vi "MeasurementSMO.TestLauncher.vi"() -> ()   [LabVIEW 2019, in "MeasurementSMO.lvclass"]
uses:
  MeasurementSMO.lvclass
  <vilib>/JKI/JKI SMO/SMO/SMO.lvclass
  <vilib>/JKI/JKI SMO/SMO/Typedefs/SMOState --Enum.ctl
  <userlib>/LevyLab/Instrument Framework/SMOs/RemoteControl/RemoteControl.lvclass
  <userlib>/LevyLab/Instrument Framework/SMOs/RemoteControl/Typedefs/RC Com Type--enum.ctl
  21cc0d15-aa5c-4e02-9f98-410864ffd08d.vi
  2cee4e23-403c-4d2f-920d-9f09caed685e.vi
  9af032d4-89d2-4663-9556-aa01e6123ab8.vi
  C:/Program Files (x86)/National Instruments/LabVIEW 2019/vi.lib/JKI/JKI SMO/SMO/SMO.lvclass
  b9372eaf-d79d-420f-ae4a-5723e45e53aa.vi
  e51c5ca0-d227-4b24-97f1-175e48e65030.vi
  Typedefs/PrivateEvents--MeasurementSMO.IV Run--Local.ctl
panel:
  in  "IV Run--Local":T1={"Pattern"=enum."Ramp /\\", "Cycles"=0.0, "Rate"=1.0, "End"=1.0, "Start"=1.0}
  out "Help Reply":string[](array[string])
  out "ACK Reply":string
  in  "HELP":bool
  in  "ACK":bool
  out "IV_ABORT Reply":string
  in  "IV_ABORT":bool
  out "IV_RUN Reply":string
  in  "IV_RUN":bool
  out "IV_Status Reply":string
  in  "IV_STATUS":bool
  out "SMO State":T2
  out "error out":errorcluster
  in  "Stop":bool
  # "Measurement SMO Test Launcher"
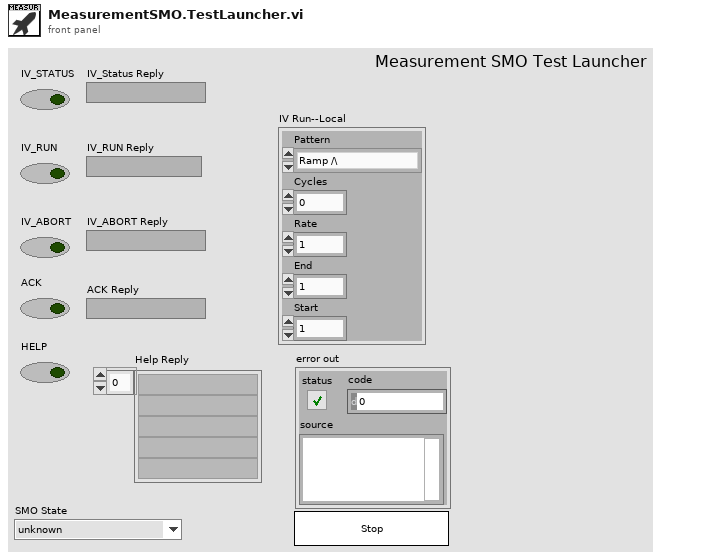
[diagram p1: front panel]
types:
  T1 = typedef "MeasurementSMO.lvclass/PrivateEvents--MeasurementSMO.IV Run--Local.ctl" = cluster{"Pattern":enum16{"Ramp /", "Ramp /\\", "Smooth Ramp _/", "Smooth Ramp _/\\_", "Frequency"}, "Cycles":dbl, "Rate":dbl, "End":dbl, "Start":dbl}
  T2 = typedef "SMO.lvclass/SMOState --Enum.ctl" = enum16{"unknown", "Created", "Started", "Stopped"}
  T3 = typedef "SMO.lvclass/Public Events.ctl" = cluster{"Error":refnum<user-event>, "State":refnum<user-event>, "Reserve State":refnum<user-event>}
  T4 = cluster{"Event Registration Refnum":refnum<event-registration>}
  T5 = typedef "RemoteControl.lvclass/RC Com Type--enum.ctl" = enum16{"RC", "STM", "ZMQ"}
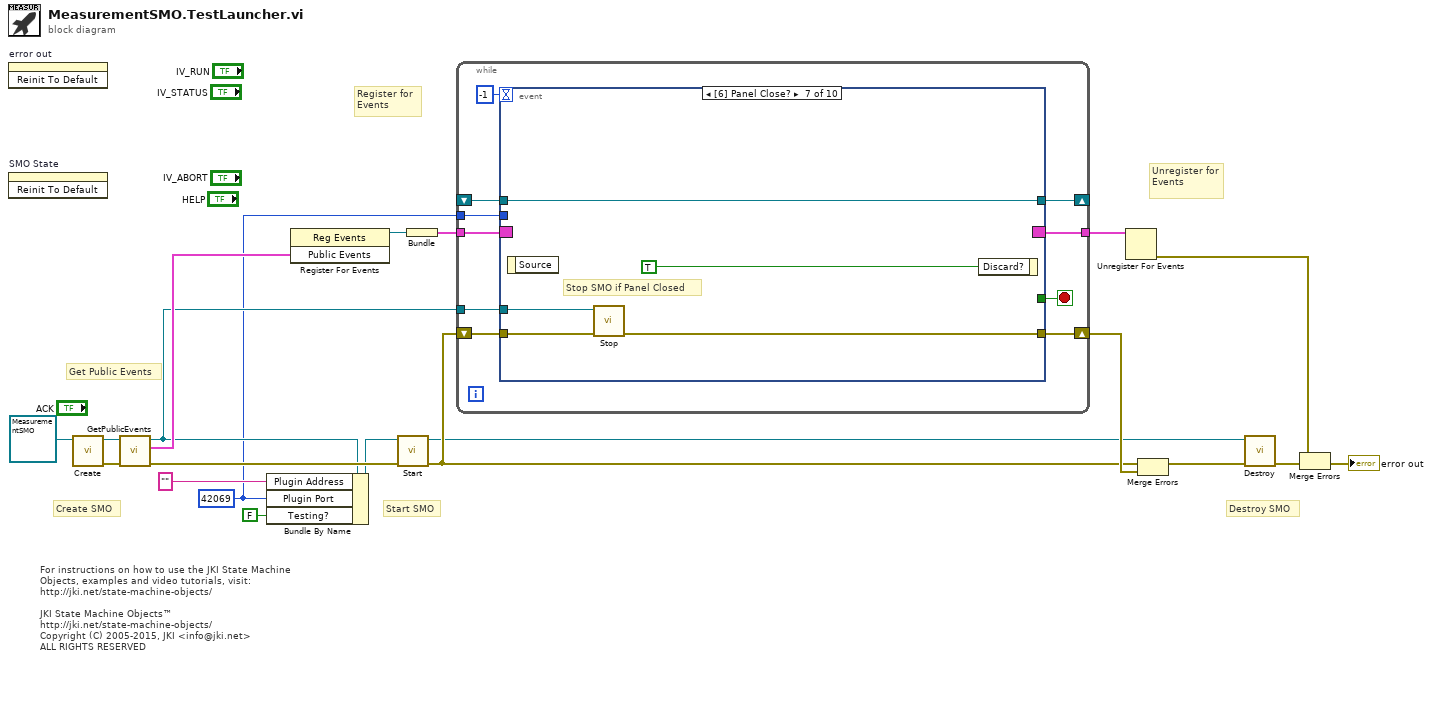
[diagram p0: block diagram]
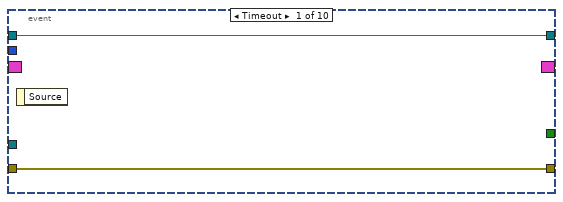
[diagram p2: hidden frame]
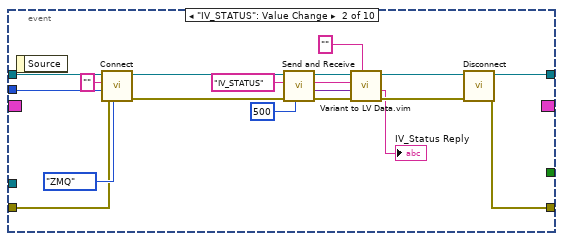
[diagram p3: hidden frame]
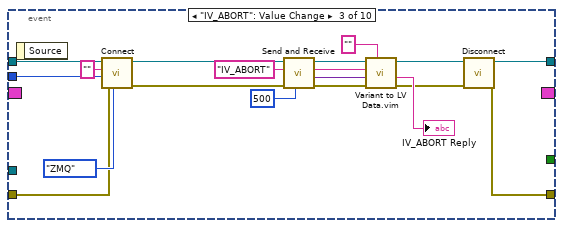
[diagram p4: hidden frame]
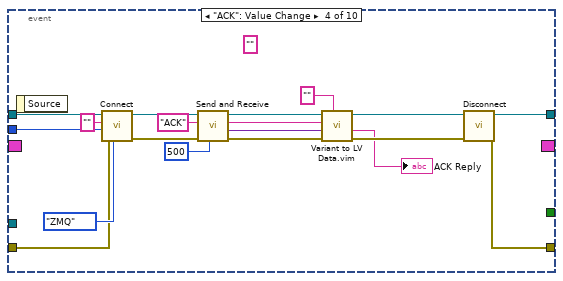
[diagram p5: hidden frame]
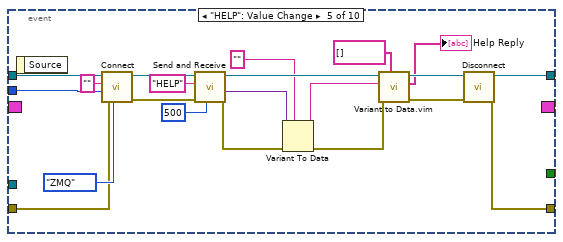
[diagram p6: hidden frame]
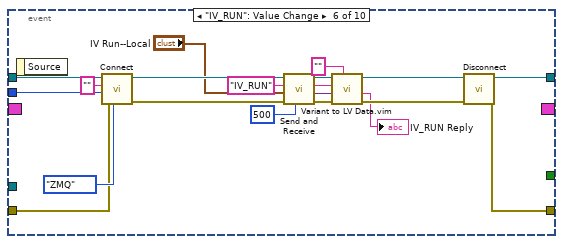
[diagram p7: hidden frame]
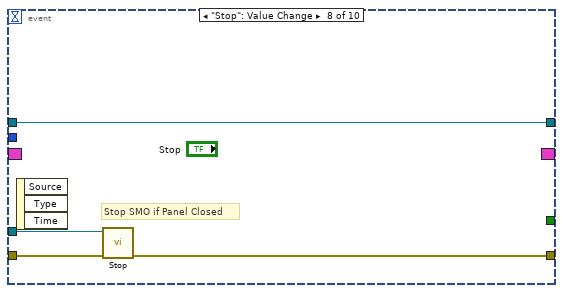
[diagram p8: hidden frame]
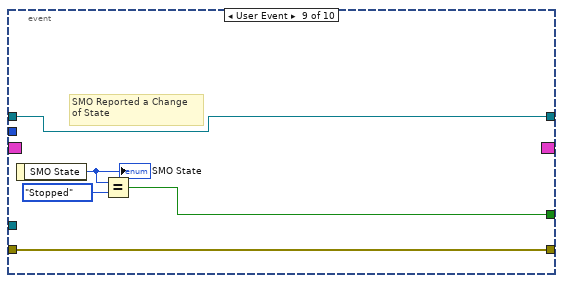
[diagram p9: hidden frame]
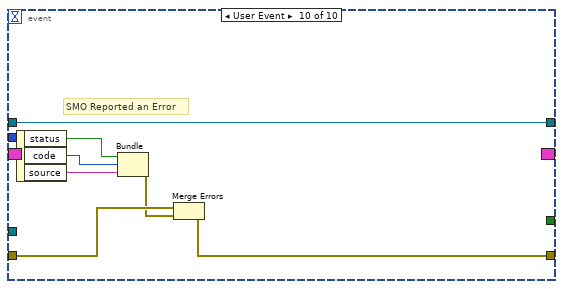
[diagram p10: hidden frame]
diagram:
  w2 = u16 42069 ("Plugin Port")
  # "For instructions on how to use the JKI State Machine Objects, examples and video tutorials, visit:\nhttp://jki.net/state-machine-objects/\n\nJKI State Machine Objects™\nhttp://jki.net/state-machine-objects/\nCopyright (C) 2005-2015, JKI <info@jki.net>\nALL RIGHTS RESERVED"
  # "Get Public Events"
  # "Start SMO"
  # "Destroy SMO"
  # "Create SMO"
  # "Unregister for Events"
  # "Register for Events"
  n1 = invoke on="error out" class="Clust (strict)" method="Reinit To Default"() -> ()  [unwired: 3 in, 3 out]
  n2 = invoke on="SMO State" class="Enum (strict)" method="Reinit To Default"() -> ()  [unwired: 3 in, 3 out]
  n3 = call <vilib>:"Create.vi"("SMO"=refnum<class "MeasurementSMO.lvclass"> refnum ("SMO.Template.lvclass")) -> ("error out"=w9:errorcluster, "SMO out"=w10:refnum<class "MeasurementSMO.lvclass">)  [unwired: 8 in, 1 out]
  n4 = call <vilib>:"GetPublicEvents.vi"("error in (no error)"=w9, "SMO"=w10) -> ("error out"=w8:errorcluster, "Public Events"=w7:T3, "SMO out"=w5:refnum<class "MeasurementSMO.lvclass">)  [unwired: 7 in]
  n5 = Bundle By Name(cluster=w5, "Plugin Address"="" ("address"), "Plugin Port"=w2, "Testing?"=FALSE) -> (w4:refnum<class "MeasurementSMO.lvclass">)
  n6 = register-events(w7) -> (reference out=w6:refnum<event-registration>)  [unwired: 2 in, 1 out]
  n7 = call <vilib>:"Start.vi"("error in (no error)"=w8, "SMO"=w4) -> ("error out"=w13:errorcluster, "SMO out"=w11:refnum<class "MeasurementSMO.lvclass">)  [unwired: 8 in]
  n8 = Bundle("Event Registration Refnum"=w6) -> (w19:T4)  [unwired: 1 in]
  n9 = while {
    shift-right: [w29] -> w18
    shift-left: w13 -> [w28]
    tunnel: w19 -> [w27]
    tunnel: [w26] -> w20
    tunnel: w5 -> [w25]
    shift-right: [w23] -> _
    shift-left: _ -> [w22]
    tunnel: w2 -> [w21]
    stop <- w30 stop-if-true
    n10 = event shown="[6] Panel Close?" {
      selector: w27 -> [_ _ _ _ _ _ _ _ _ _]
      dyn-events: [_ _ _ _ _ _ _ _ _ _] -> w26
      timeout: -1 -> [_ _ _ _ _ _ _ _ _ _]
      tunnel: [_ _ _ _ _ _ _ _ w137 _] -> w30
      tunnel: w25 -> [_ _ _ _ _ _ w131 w135 _ _]
      tunnel: [w32 w45 w63 w82 w103 w121 w130 w134 w140 w145] -> w29
      tunnel: w28 -> [w32 w44 w62 w81 w102 w120 w129 w133 w140 w143]
      tunnel: [w31 w41 w59 w78 w99 w117 w127 w132 w136 w141] -> w23
      tunnel: w22 -> [w31 w40 w58 w77 w98 w116 w127 w132 w136 w141]
      tunnel: w21 -> [_ w33 w51 w69 w87 w108 _ _ _ _]
      event Timeout {
        n11 = event-data() -> ()  [unwired: 1 in, 1 out]
      }
      event "IV_STATUS": Value Change {
        n12 = event-data() -> ()  [unwired: 1 in, 1 out]
        n13 = call <userlib>:"Connect.vi"("RC Type"=RC_Com_Type--enum."ZMQ", "error in (no error)"=w44, "Port"=w33, "address"="", "RemoteControl in"=w40) -> ("error out"=w46:errorcluster, "RemoteControl out"=w50:refnum<class "RemoteControl.lvclass">)  [unwired: 5 in]
        n14 = call <userlib>:"Send and Receive.vi"("timeout (ms) [500]"=500, "error in (no error)"=w46, "Command"="IV_STATUS", "RemoteControl in"=w50) -> ("error out"=w39:errorcluster, "Data out"=w35:variant, "Command out"=w36:string, "RemoteControl out"=w49:refnum<class "RemoteControl.lvclass">)  [unwired: 4 in]
        n15 = call "Variant to LV Data.vim"("type"="", "error in (no error)"=w39, "JSON Data in"=w35, "Command"=w36) -> ("error out"=w38:errorcluster, "Data out"=→"IV_Status Reply":string)  [unwired: 4 in, 2 out]
        n16 = call <userlib>:"Disconnect.vi"("error in (no error)"=w38, "RemoteControl in"=w49) -> ("error out"=w45:errorcluster, "RemoteControl out"=w41:refnum<class "RemoteControl.lvclass">)  [unwired: 8 in]
      }
      event "IV_ABORT": Value Change {
        n17 = event-data() -> ()  [unwired: 1 in, 1 out]
        n18 = call <userlib>:"Connect.vi"("RC Type"=RC_Com_Type--enum."ZMQ", "error in (no error)"=w62, "Port"=w51, "address"="", "RemoteControl in"=w58) -> ("error out"=w64:errorcluster, "RemoteControl out"=w68:refnum<class "RemoteControl.lvclass">)  [unwired: 5 in]
        n19 = call <userlib>:"Send and Receive.vi"("timeout (ms) [500]"=500, "error in (no error)"=w64, "Command"="IV_ABORT", "RemoteControl in"=w68) -> ("error out"=w54:errorcluster, "Data out"=w57:variant, "Command out"=w56:string, "RemoteControl out"=w67:refnum<class "RemoteControl.lvclass">)  [unwired: 4 in]
        n20 = call "Variant to LV Data.vim"("type"="", "error in (no error)"=w54, "JSON Data in"=w57, "Command"=w56) -> ("error out"=w52:errorcluster, "Data out"=→"IV_ABORT Reply":string)  [unwired: 4 in, 2 out]
        n21 = call <userlib>:"Disconnect.vi"("error in (no error)"=w52, "RemoteControl in"=w67) -> ("error out"=w63:errorcluster, "RemoteControl out"=w59:refnum<class "RemoteControl.lvclass">)  [unwired: 8 in]
      }
      event "ACK": Value Change {
        (unwired) ""
        n22 = event-data() -> ()  [unwired: 1 in, 1 out]
        n23 = call <userlib>:"Connect.vi"("RC Type"=RC_Com_Type--enum."ZMQ", "error in (no error)"=w81, "Port"=w69, "address"="", "RemoteControl in"=w77) -> ("error out"=w83:errorcluster, "RemoteControl out"=w86:refnum<class "RemoteControl.lvclass">)  [unwired: 5 in]
        n24 = call <userlib>:"Send and Receive.vi"("timeout (ms) [500]"=500, "error in (no error)"=w83, "Command"="ACK", "RemoteControl in"=w86) -> ("error out"=w76:errorcluster, "Data out"=w74:variant, "Command out"=w73:string, "RemoteControl out"=w70:refnum<class "RemoteControl.lvclass">)  [unwired: 4 in]
        n25 = call "Variant to LV Data.vim"("type"="", "error in (no error)"=w76, "JSON Data in"=w74, "Command"=w73) -> ("error out"=w75:errorcluster, "Data out"=→"ACK Reply":string)  [unwired: 4 in, 2 out]
        n26 = call <userlib>:"Disconnect.vi"("error in (no error)"=w75, "RemoteControl in"=w70) -> ("error out"=w82:errorcluster, "RemoteControl out"=w78:refnum<class "RemoteControl.lvclass">)  [unwired: 8 in]
      }
      event "HELP": Value Change {
        n27 = event-data() -> ()  [unwired: 1 in, 1 out]
        n28 = call <userlib>:"Connect.vi"("RC Type"=RC_Com_Type--enum."ZMQ", "error in (no error)"=w102, "Port"=w87, "address"="", "RemoteControl in"=w98) -> ("error out"=w104:errorcluster, "RemoteControl out"=w107:refnum<class "RemoteControl.lvclass">)  [unwired: 5 in]
        n29 = call <userlib>:"Send and Receive.vi"("timeout (ms) [500]"=500, "error in (no error)"=w104, "Command"="HELP", "RemoteControl in"=w107) -> ("error out"=w92:errorcluster, "Data out"=w88:variant, "RemoteControl out"=w96:refnum<class "RemoteControl.lvclass">)  [unwired: 4 in, 1 out]
        n30 = Variant To Data(error in=w92, type="", Variant=w88) -> (data=w89:string, error out=w91:errorcluster)
        n31 = call "Variant to Data.vim"("Data Type"=string[] [], "error in (no error)"=w91, "Data in"=w89, "RemoteControl in"=w96) -> ("error out"=w90:errorcluster, "Data out"=→"Help Reply":string[], "RemoteControl out"=w97:refnum<class "RemoteControl.lvclass">)  [unwired: 5 in]
        n32 = call <userlib>:"Disconnect.vi"("error in (no error)"=w90, "RemoteControl in"=w97) -> ("error out"=w103:errorcluster, "RemoteControl out"=w99:refnum<class "RemoteControl.lvclass">)  [unwired: 8 in]
      }
      event "IV_RUN": Value Change {
        n33 = event-data() -> ()  [unwired: 1 in, 1 out]
        n34 = call <userlib>:"Connect.vi"("RC Type"=RC_Com_Type--enum."ZMQ", "error in (no error)"=w120, "Port"=w108, "address"="", "RemoteControl in"=w116) -> ("error out"=w122:errorcluster, "RemoteControl out"=w126:refnum<class "RemoteControl.lvclass">)  [unwired: 5 in]
        n35 = call <userlib>:"Send and Receive.vi"("timeout (ms) [500]"=500, "error in (no error)"=w122, "Data"="IV Run--Local", "Command"="IV_RUN", "RemoteControl in"=w126) -> ("error out"=w114:errorcluster, "Data out"=w112:variant, "Command out"=w111:string, "RemoteControl out"=w125:refnum<class "RemoteControl.lvclass">)  [unwired: 3 in]
        n36 = call "Variant to LV Data.vim"("type"="", "error in (no error)"=w114, "JSON Data in"=w112, "Command"=w111) -> ("error out"=w113:errorcluster, "Data out"=→"IV_RUN Reply":string)  [unwired: 4 in, 2 out]
        n37 = call <userlib>:"Disconnect.vi"("error in (no error)"=w113, "RemoteControl in"=w125) -> ("error out"=w121:errorcluster, "RemoteControl out"=w117:refnum<class "RemoteControl.lvclass">)  [unwired: 8 in]
      }
      event Panel Close? {
        # "Stop SMO if Panel Closed"
        n38 = event-data() -> ()  [unwired: 1 in, 1 out]
        n39 = call <vilib>:"Stop.vi"("error in (no error)"=w129, "SMO"=w131) -> ("error out"=w130:errorcluster)  [unwired: 8 in, 1 out]
        n40 = event-data("Discard?"=TRUE ("OK")) -> ()  [unwired: 1 in, 1 out]
      }
      event "Stop": Value Change {
        # "Stop SMO if Panel Closed"
        n41 = event-data() -> ()  [unwired: 1 in, 3 out]
        n42 = call <vilib>:"Stop.vi"("error in (no error)"=w133, "SMO"=w135) -> ("error out"=w134:errorcluster)  [unwired: 8 in, 1 out]
      }
      event User Event {
        # "SMO Reported a Change\nof State"
        n43 = event-data() -> ("SMO State"=w139:T2)  [unwired: 1 in]
        "SMO State" <- w139
        n44 = Equal?(x=w139, y=SMOState_--Enum."Stopped") -> (x = y?=w137:bool)
      }
      event User Event {
        # "SMO Reported an Error"
        n45 = event-data() -> ("status"=w144:bool, "code"=w147:i32, "source"=w146:string)  [unwired: 1 in]
        n46 = Bundle("status"=w144, "code"=w147, "source"=w146) -> (w142:errorcluster)  [unwired: 1 in]
        n47 = Merge Errors(w143, w142) -> (w145:errorcluster)
      }
    }
  }
  n48 = Unregister For Events(event registration refnum=w20) -> (error out=w17:errorcluster)  [unwired: 1 in]
  n49 = Merge Errors(w13, w18) -> (w12:errorcluster)
  n50 = call <vilib>:"Destroy.vi"("error in (no error)"=w12, "SMO"=w11) -> ("error out"=w15:errorcluster)  [unwired: 9 in]
  n51 = Merge Errors(w17, w15) -> (→"error out":errorcluster)
